vi "CoolLED.vi"() -> ()   [LabVIEW 2025]
panel:
  in  "Stop":bool
  in  "Store":bool
  in  "Presets":enum16{"DAPI", "GFP", "RFP", "None", "Multiple"}(ring)=enum."None"
  in  "Cluster":T1 {"Green-Red" step=1 scale=0.0..100.0; "Blue" step=1 scale=0.0..100.0; "Violet" step=1 scale=0.0..100.0}
  out "error out":errorcluster
  in  "error in":errorcluster
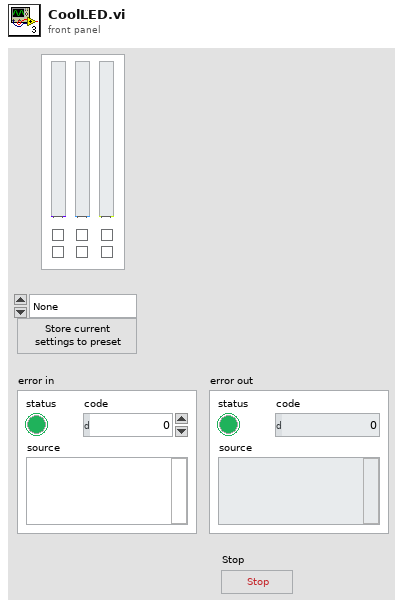
[diagram p1: front panel]
types:
  T1 = cluster{"Violet":u8, "Blue":u8, "Green-Red":u8, "A(S)Selected/(N)Unselected":bool, "B(S)Selected/(N)Unselected":bool, "C(S)Selected/(N)Unselected":bool, "A(N)ON/(F)OFF":bool, "(N)ON/(F)OFF":bool, "C(N)ON/(F)OFF":bool}
  T2 = typedef "Message Queue.lvlib/All Message Queues.ctl" = cluster{"CoolLED":refnum<queue>}
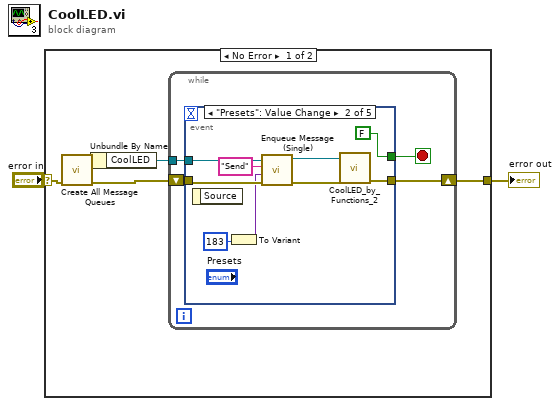
[diagram p0: block diagram]
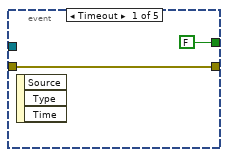
[diagram p2: hidden frame]
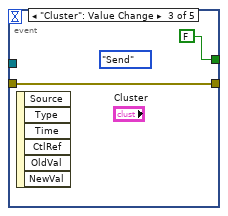
[diagram p3: hidden frame]
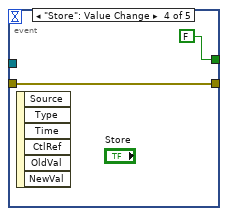
[diagram p4: hidden frame]
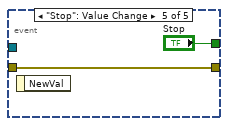
[diagram p5: hidden frame]
diagram:
  n1 = case shown="No Error" "error in" {
    selector: "error in" -> [w6 w29]
    tunnel: [w7 w29] -> w1
    frame No Error {
      n2 = call "Create All Message Queues.vi"("error in (no error)"=w6) -> ("error out"=w5:errorcluster, "Message Queues out"=w4:T2)  [unwired: 9 in]
      n3 = Unbundle By Name(w4) -> ("CoolLED"=w3:refnum<queue>)
      n4 = while {
        shift-right: [w10] -> w7
        shift-left: w5 -> [w11]
        tunnel: w3 -> [w8]
        stop <- w9 stop-if-true
        n5 = event shown="[1] \"Presets\": Value Change" {
          selector: _ -> [_ _ _ _ _]
          dyn-events: _ -> [_ _ _ _ _]
          timeout: _ -> [_ _ _ _ _]
          tunnel: w11 -> [w13 w19 w23 w26 w27]
          tunnel: [w13 w22 w23 w26 w27] -> w10
          tunnel: [FALSE ("Stop") FALSE ("Stop") FALSE ("Stop") FALSE ("Stop") "Stop"] -> w9
          tunnel: w8 -> [_ w20 _ _ _]
          event Timeout {
            n6 = event-data() -> ()  [unwired: 1 in, 3 out]
          }
          event "Presets": Value Change {
            n7 = event-data() -> ()  [unwired: 1 in, 1 out]
            n8 = To Variant(anything=u8 183) -> (Variant=w17:variant)
            n9 = call "Enqueue Message (Single).vi"("error in (no error)"=w19, "Message Data"=w17, "Message"="Send", "Message Queue"=w20) -> ("error out"=w15:errorcluster, "dup Message Queue"=w14:refnum<queue>)  [unwired: 6 in]
            n10 = call "CoolLED_by_Functions_2.vi"("error in (no error)"=w15, "Message Queue"=w14) -> ("error out"=w22:errorcluster)  [unwired: 9 in]
          }
          event "Cluster": Value Change {
            (unwired) enum16{"Initialize", "Send", "Store", "Close"}."Send" ("Function")
            n11 = event-data() -> ()  [unwired: 1 in, 6 out]
          }
          event "Store": Value Change {
            n12 = event-data() -> ()  [unwired: 1 in, 6 out]
          }
          event "Stop": Value Change {
            n13 = event-data() -> ()  [unwired: 1 in, 1 out]
          }
        }
      }
    }
    frame Error {
    }
  }
  "error out" <- w1
